vi "FPGA_main.vi"() -> ()   [LabVIEW 2019]
uses:
  #typedef_FPGA_States.ctl
  <vilib>/Platform/TimedLoop/XDataNode/timing_clust.ctl
  <vilib>/Platform/TimedLoop/XDataNode/nitl_modes.ctl
  <vilib>/Platform/TimedLoop/XDataNode/wakeup.ctl
  <vilib>/rvi/Emulation/niFpgaGetClockAttributes.vi
  <vilib>/rvi/Emulation/niFpgaSctlEmulationGetInTimedLoop.vi
  <vilib>/rvi/Emulation/niFpgaEmulationReportErrorSimple.vi
  <vilib>/rvi/eio/common/nirviEmuTemplateMethod_errors.vi
  <vilib>/rvi/Emulation/niFpgaEmulationIsFPGAContextNoSignature.vi
  <vilib>/rvi/DataTransferAndStorage/Container/Common/niFpgaContainerGetUniqueNameForEmu.vi
  <vilib>/rvi/Memory/Memory_Emulation/niFpgaMemoryEmulationCacheClearOnFirstRun.vi
  <vilib>/rvi/Memory/Memory_Emulation/nirvimemoryEmulationManagerCache_MakeExclusive.vi
  <vilib>/rvi/Memory/Memory_Emulation/niFpgaMemoryEmulationValidateCache.vi
  <vilib>/rvi/Memory/Memory_Emulation/nirvimemoryEmulationManagerCache_InsertValue.vi
  <vilib>/Utility/error.llb/Clear Errors.vi
  <vilib>/rvi/Memory/Memory_Emulation/nirvimemoryEmulationManagerCache_ReleaseExclusive.vi
  <vilib>/rvi/Memory/Memory_Emulation/nirvimemoryEmulationManagerCache_GetValue.vi
  <vilib>/rvi/Memory/Memory_Emulation/nirvimemoryEmulationManagerCache_SetValue.vi
  <vilib>/rvi/Emulation/niFpgaProcessEmulError.vi
  <vilib>/rvi/Emulation/niFpgaCriticalErrorInLSC.vi
  <vilib>/rvi/errors/niFpgaSetErrorForExecOnDevCompSimple.vi
  <vilib>/rvi/eio/common/nirviEmuReportErrorAndStop.vi
  <vilib>/rvi/FIFO/Fifo_Resource/nirvififoEmulationSetSize.vi
  <vilib>/rvi/FIFO/Fifo_Resource/nirviFifoEmulationQueueMgr.vi
  <instcachedir>/0/nirviFifoEmulationQueueMgr_E5CAEC123FF24DC58D834DCA3CDAA9B5.lvgen/nirviFifoEmulationQueueMgr_E5CAEC123FF24DC58D834DCA3CDAA9B5_002.vi
  <vilib>/rvi/FIFO/Fifo_Resource/nirvififoEmulationDetermineInputValidOut.vi
  <vilib>/rvi/FIFO/Fifo_Resource/nirvififoEmulationCreateLock.vi
  <vilib>/rvi/FIFO/Fifo_Resource/nirvififoEmulationObtainLock.vi
  <vilib>/rvi/FIFO/Fifo_Resource/nirvififoEmulationReleaseLock.vi
  <vilib>/rvi/occurrence/nirviWaitOnOccurrenceBase.vi
  <vilib>/rvi/errors/nirviReportUnexpectedCaseInternalError.vi
  <vilib>/rvi/errors/nirviReportUnexpectedCaseInternalError (U32).vi
  <vilib>/rvi/Memory/Memory_Emulation/nirvimemoryFastEmulation.vi
  <vilib>/rvi/Memory/Memory_Emulation/nirvimemoryEmulation.vi
  <vilib>/rvi/interface/RandomDataEmulation/niFpgaRandomDataHandleErrors.vi
  <vilib>/eio/EIONode/EIONode.xnode
  <vilib>/rvi/DataTransferAndStorage/Container/XNode/niFpgaContainer.xnode
  <vilib>/rvi/DataTransferAndStorage/Register/Emulation/niFpgaRegisterEmulation.vi
  <vilib>/platform/TimedLoop/XDataNode/XDataNode.xnode
  <vilib>/rvi/FIFO/Fifo_Resource/nirvififoEmulationWrite.vi
  <vilib>/rvi/DataTransferAndStorage/Handshake/Emulation/niFpgaHandshakeEmulation.vi
  <vilib>/rvi/FIFO/Fifo_Resource/nirvififoEmulationRead.vi
  <vilib>/rvi/interface/RandomDataEmulation/nirviRandomDataFpgaReadWriteTemplate.vi
  <vilib>/Platform/TimedLoop/XDataNode/XDNodeRunTimeDep.lvlib
panel:
  out "Data":u32
  in  "PosttriggerLenght":u16
  in  "PretriggerLenght":u16
  in  "Monitoring?":bool
  in  "stop":bool
  in  "TriggerZ":i16
  in  "TriggerY":i16
  in  "SamplesOverTreshold":u8
  in  "TriggerX":i16
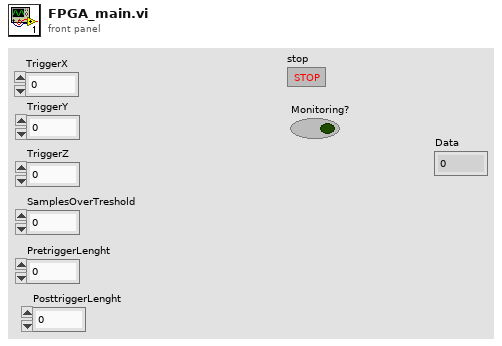
[diagram p1: front panel]
types:
  T1 = typedef "#typedef_FPGA_States.ctl" = enum16{"Idle", "Monitoring", "SendPretriggerData", "SendPostriggerData"}
  T2 = typedef "XDNodeRunTimeDep.lvlib/timing_clust.ctl" = cluster{"Expected End [f-1]":u64, "Actual End [f-1]":u64, "Finished Late? [f-1]":bool, "Expected End [i-1]":u64, "Actual End [i-1]":u64, "Finished Late? [i-1]":bool, "Expected Start [i]":u64, "Actual Start [i]":u64, "Expected Start [f]":u64, "Actual Start [f]":u64, "Source Name":string, "Structure Name":string, "Period":i64, "Deadline":i64, "Offset":i64, "Start":i64, "Priority":i32, "Timeout":i32, "Mode":T3, "Wakeup Reason":T4, "Error":errorcluster, "Source Type":string, "Secondary Source Type":string, "Global End Time":u64, "Global Start Time":u64, "Frame Duration":u64, "Iteration Duration":u64, "Assigned CPU":i32, "I/O Scan Engine Mode":u32}
  T3 = typedef "XDNodeRunTimeDep.lvlib/nitl_modes.ctl" = enum32{"No Change", "Process missed periods, maintain original phase", "Discard missed periods, maintain original phase", "Process missed periods, ignore original phase", "Discard missed periods, ignore original phase"}
  T4 = typedef "XDNodeRunTimeDep.lvlib/wakeup.ctl" = enum32{"Normal", "Aborted", "Asynchronous wakeup", "Timing source error", "Timed loop error", "Timeout"}
  T5 = cluster{"AccelerationX":i16, "AccelerationY":i16, "AccelerationZ":i16}
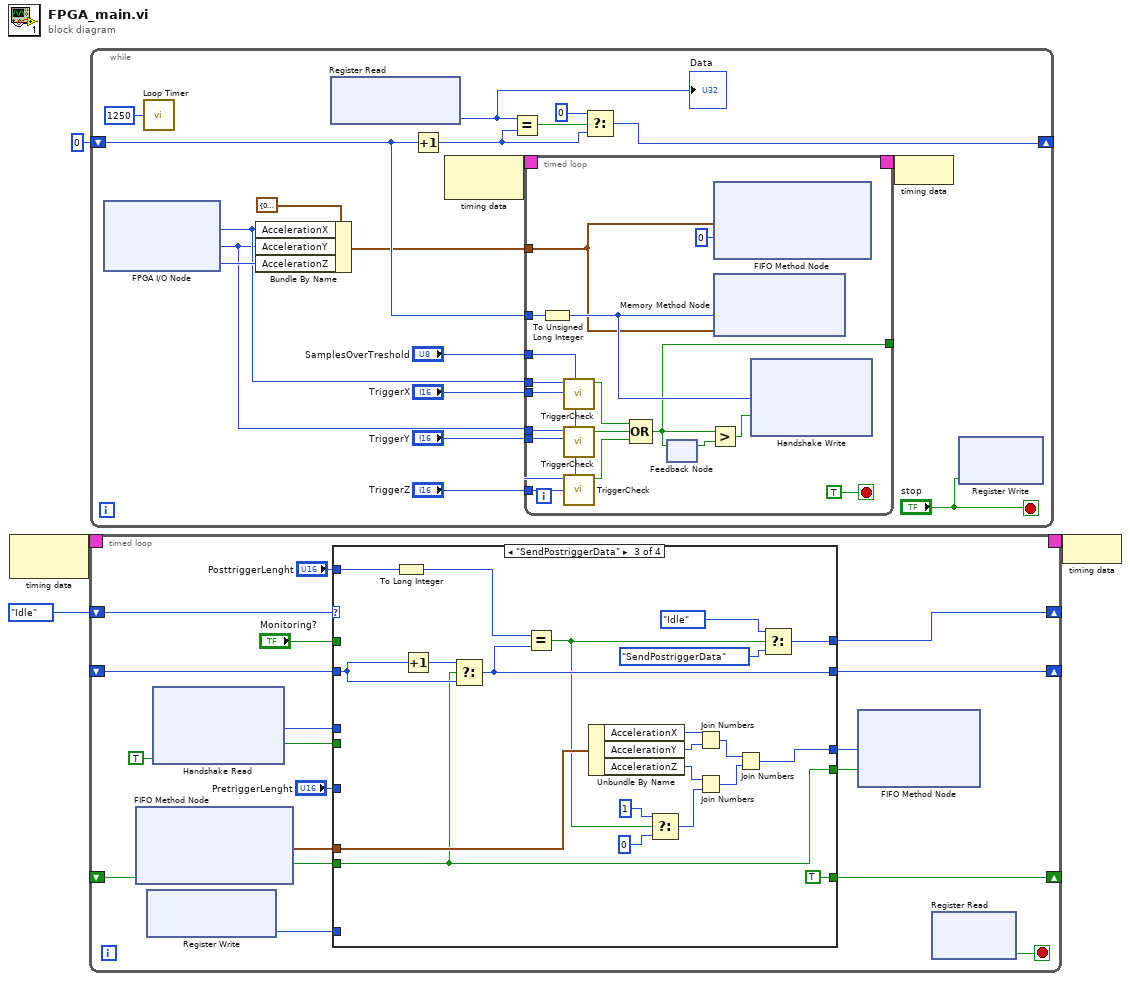
[diagram p0: block diagram]
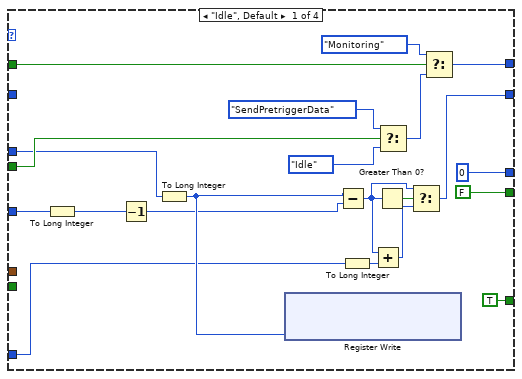
[diagram p2: hidden frame]
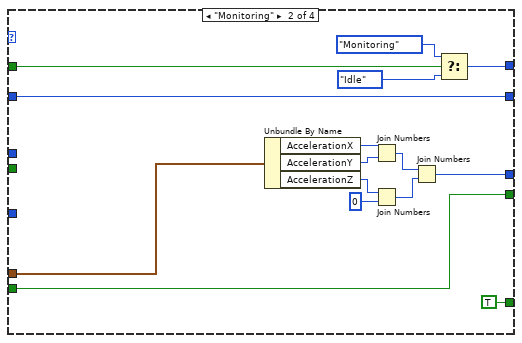
[diagram p3: hidden frame]
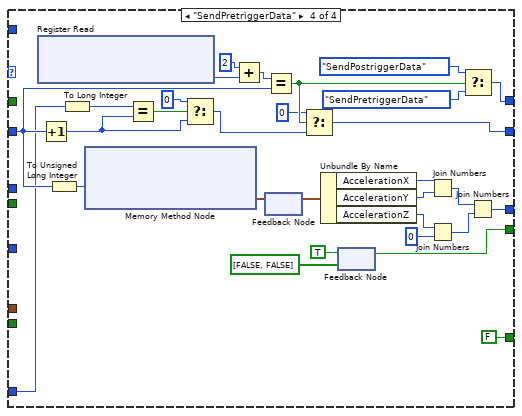
[diagram p4: hidden frame]
diagram:
  n1 = node-c288() -> (w3:T2)  [unwired: 1 in]
  n2 = timed-loop {
    timing: w3 -> [_]
    timing-out: [_] -> w2
    shift-right: [w21] -> _
    shift-left: #typedef_FPGA_States."Idle" ("FPGA States") -> [w22]
    shift-right: [w15] -> _
    shift-left: _ -> [w16]
    shift-right: [w10] -> _
    shift-left: _ -> [w11]
    stop <- w17 stop-if-true
    n3 = xnode ("FIFO Method Node")("Ready for Output"=w11) -> ("Element"=w12:T5, "Output Valid"=w9:bool)  [unwired: 1 in, 1 out]
    n4 = xnode "Register Write"() -> ("Data"=w5:u32)  [unwired: 1 in, 1 out]
    n5 = xnode ("Handshake Read")("Ready for Output"=TRUE) -> ("Data"=w6:u32, "Output Valid"=w7:bool)  [unwired: 1 in, 1 out]
    n6 = case shown="\"SendPostriggerData\"" w22 {
      tunnel: [w43 w48 w70 w99] -> w21
      tunnel: [u64 0 ("Element") w49 w71 w101] -> w20
      tunnel: [FALSE ("Input Valid") w45 w62 w88] -> w19
      tunnel: "Monitoring?" -> [w36 w57 _ _]
      tunnel: w16 -> [_ w47 w63 w97]
      tunnel: [w27 w47 w64 w84] -> w15
      tunnel: "PretriggerLenght" -> [w35 _ _ _]
      tunnel: "PosttriggerLenght" -> [_ _ w69 _]
      tunnel: w12 -> [_ w46 w66 _]
      tunnel: w9 -> [_ w45 w62 _]
      tunnel: [TRUE TRUE TRUE FALSE] -> w10
      tunnel: w7 -> [w32 _ _ _]
      tunnel: w6 -> [w31 _ _ _]
      tunnel: w5 -> [w23 _ _ w81]
      frame "Idle", Default {
        n7 = To Long Integer(number=w35) -> (32bit integer=w34:i32)
        n8 = Decrement(x=w34) -> (x-1=w25:i32)
        n9 = To Long Integer(number=w31) -> (32bit integer=w26:i32)
        n10 = xnode ("Register Write")("Data"=w26) -> ()  [unwired: 1 in, 1 out]
        n11 = Subtract(x=w26, y=w25) -> (x-y=w30:i32)
        n12 = To Long Integer(number=w23) -> (32bit integer=w24:i32)
        n13 = Add(x=w30, y=w24) -> (x+y=w29:i32)
        n14 = Greater Than 0?(x=w30) -> (x > 0?=w28:bool)
        n15 = Select(t=#typedef_FPGA_States."SendPretriggerData" ("FPGA States"), s=w32, f=#typedef_FPGA_States."Idle" ("FPGA States")) -> (s? t:f=w41:T1)
        n16 = Select(t=w30, s=w28, f=w29) -> (s? t:f=w27:i32)
        n17 = Select(t=#typedef_FPGA_States."Monitoring" ("FPGA States"), s=w36, f=w41) -> (s? t:f=w43:T1)
      }
      frame "Monitoring" {
        n18 = Unbundle By Name(w46) -> ("AccelerationX"=w55:i16, "AccelerationY"=w54:i16, "AccelerationZ"=w53:i16)
        n19 = Join Numbers(hi=w55, lo=w54) -> ((hi.lo)=w51:u32)
        n20 = Join Numbers(hi=w53, lo=i16 0) -> ((hi.lo)=w50:u32)
        n21 = Join Numbers(hi=w51, lo=w50) -> ((hi.lo)=w49:u64)
        n22 = Select(t=#typedef_FPGA_States."Monitoring" ("FPGA States"), s=w57, f=#typedef_FPGA_States."Idle" ("FPGA States")) -> (s? t:f=w48:T1)
      }
      frame "SendPostriggerData" {
        n23 = To Long Integer(number=w69) -> (32bit integer=w68:i32)
        n24 = Increment(x=w63) -> (x+1=w67:i32)
        n25 = Select(t=w67, s=w62, f=w63) -> (s? t:f=w64:i32)
        n26 = Equal?(x=w68, y=w64) -> (x = y?=w60:bool)
        n27 = Unbundle By Name(w66) -> ("AccelerationX"=w77:i16, "AccelerationY"=w76:i16, "AccelerationZ"=w75:i16)
        n28 = Select(t=i16 1, s=w60, f=i16 0 ("lo")) -> (s? t:f=w61:i16)
        n29 = Join Numbers(hi=w77, lo=w76) -> ((hi.lo)=w73:u32)
        n30 = Join Numbers(hi=w75, lo=w61) -> ((hi.lo)=w72:u32)
        n31 = Join Numbers(hi=w73, lo=w72) -> ((hi.lo)=w71:u64)
        n32 = Select(t=#typedef_FPGA_States."Idle" ("FPGA States"), s=w60, f=#typedef_FPGA_States."SendPostriggerData" ("FPGA States")) -> (s? t:f=w70:T1)
      }
      frame "SendPretriggerData" {
        n33 = xnode ("Register Read")() -> ("Data"=w92:i32)  [unwired: 1 in, 1 out]
        n34 = Increment(x=w97) -> (x+1=w95:i32)
        n35 = To Unsigned Long Integer(number=w97) -> (unsigned 32bit integer=w98:u32)
        n36 = To Long Integer(number=w81) -> (32bit integer=w80:i32)
        n37 = xnode ("Memory Method Node")("Address"=w98) -> ("Data"=w100:T5)  [unwired: 1 in, 1 out]
        n38 = Equal?(x=w80, y=w95) -> (x = y?=w96:bool)
        n39 = Select(t=0, s=w96, f=w95) -> (s? t:f=w94:i32)
        n40 = Add(x=2, y=w92) -> (x+y=w87:i32)
        n41 = feedback-in #1(w100) -> ()
        n42 = feedback #1() -> (w91:T5)  [unwired: 1 in]
        n43 = Equal?(x=w87, y=w97) -> (x = y?=w83:bool)
        n44 = Select(t=0, s=w83, f=w94) -> (s? t:f=w84:i32)
        n45 = Unbundle By Name(w91) -> ("AccelerationX"=w107:i16, "AccelerationY"=w106:i16, "AccelerationZ"=w105:i16)
        n46 = feedback #2(bool[] [FALSE, FALSE]) -> (w88:bool)
        n47 = feedback-in #2(TRUE) -> ()
        n48 = Join Numbers(hi=w107, lo=w106) -> ((hi.lo)=w103:u32)
        n49 = Join Numbers(hi=w105, lo=i16 0) -> ((hi.lo)=w102:u32)
        n50 = Select(t=#typedef_FPGA_States."SendPostriggerData" ("FPGA States"), s=w83, f=#typedef_FPGA_States."SendPretriggerData" ("FPGA States")) -> (s? t:f=w99:T1)
        n51 = Join Numbers(hi=w103, lo=w102) -> ((hi.lo)=w101:u64)
      }
    }
    n52 = xnode ("FIFO Method Node")("Element"=w20, "Input Valid"=w19) -> ()  [unwired: 1 in, 2 out]
    n53 = xnode ("Register Read")() -> ("Data"=w17:bool)  [unwired: 1 in, 1 out]
  }
  n54 = while {
    shift-right: [w124] -> _
    shift-left: u32 0 ("x") -> [w123]
    stop <- "stop" stop-if-true
    n55 = xnode "FPGA I/O Node"() -> ("AccelerationX"=w121:i16, "AccelerationY"=w120:i16, "AccelerationZ"=w129:i16)  [unwired: 3 in, 3 out]
    n56 = call "Loop Timer"("Count(uSec)"=u16 1250) -> ()  [unwired: 1 out]
    n57 = Bundle By Name(cluster=T5 {"AccelerationX"=0, "AccelerationY"=0, "AccelerationZ"=0} ("Data"), "AccelerationX"=w121, "AccelerationY"=w120, "AccelerationZ"=w129) -> (w116:T5)
    n58 = xnode "Register Read"() -> ("Data"=w112:u32)  [unwired: 1 in, 1 out]
    "Data" <- w112
    n59 = Increment(x=w123) -> (x+1=w125:u32)
    n60 = node-c288() -> (w114:T2)  [unwired: 1 in]
    n61 = Equal?(x=w112, y=w125) -> (x = y?=w127:bool)
    n62 = timed-loop {
      timing: w114 -> [_]
      timing-out: [_] -> w113
      tunnel: w123 -> [w147]
      tunnel: "SamplesOverTreshold" -> [w146]
      tunnel: w121 -> [w145]
      tunnel: w120 -> [w144]
      tunnel: "TriggerX" -> [w143]
      tunnel: "TriggerY" -> [w142]
      tunnel: "TriggerZ" -> [w141]
      tunnel: w116 -> [w132]
      tunnel: [w133] -> _
      stop <- TRUE stop-if-true
      n63 = To Unsigned Long Integer(number=w147) -> (unsigned 32bit integer=w134:u32)
      n64 = call "TriggerCheck.vi"("SamplesOverThreshold"=w146, "TriggerLevel"=w143, "Acceleration"=w145) -> ("Trigger?"=w140:bool)  [unwired: 8 in]
      n65 = call "TriggerCheck.vi"("SamplesOverThreshold"=w146, "TriggerLevel"=w142, "Acceleration"=w144) -> ("Trigger?"=w139:bool)  [unwired: 8 in]
      n66 = call "TriggerCheck.vi"("SamplesOverThreshold"=w146, "TriggerLevel"=w141, "Acceleration"=w144) -> ("Trigger?"=w138:bool)  [unwired: 8 in]
      n67 = Compound Arithmetic op=OR(w140, w139, w138) -> (w133:bool)
      n68 = feedback-in #3(w133) -> ()
      n69 = feedback #3() -> (w136:bool)  [unwired: 1 in]
      n70 = Greater?(x=w133, y=w136) -> (0:w135:bool)
      n71 = xnode ("FIFO Method Node")("Element"=w132, "Timeout"=0) -> ()  [unwired: 1 in, 2 out]
      n72 = xnode ("Memory Method Node")("Address"=w134, "Data"=w132) -> ()  [unwired: 1 in, 1 out]
      n73 = xnode ("Handshake Write")("Data"=w134, "Input Valid"=w135) -> ()  [unwired: 1 in, 2 out]
    }
    n74 = Select(t=u32 0 ("x"), s=w127, f=w125) -> (s? t:f=w124:u32)
    n75 = node-c288(w113) -> ()
    n76 = xnode ("Register Write")("Data"="stop") -> ()  [unwired: 1 in, 1 out]
  }
  n77 = node-c288(w2) -> ()
